vi "Read Pages.vi"(9 "PageSelector in":refnum<class "PageSelector.lvclass">) -> (3 "PageSelector out":refnum<class "PageSelector.lvclass">, 4 "Pages":refnum<class "Page.lvclass">[](array[class]))   [LabVIEW 2014, in "PageSelector.lvclass"]
uses:
  PageSelector.lvclass
  Page/Page.lvclass
  PageSelector.lvclass/PageSelector.ctl
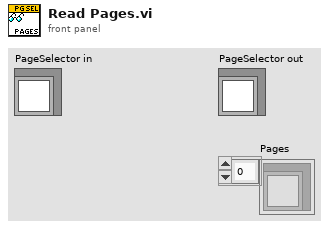
[diagram p1: front panel]
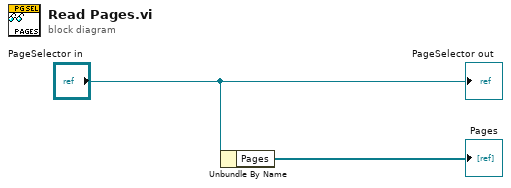
[diagram p0: block diagram]
diagram:
  n1 = Unbundle By Name("PageSelector in") -> ("Pages"=→"Pages":refnum<class "Page.lvclass">[])
  "PageSelector out" <- "PageSelector in"
